vi "Build_footer_text.vi"(4 "Invalid line":string, 6 "Error string":string, 9 "Run time":dbl, 10 "Start time":timestamp, 11 "File Text":string) -> (3 "file w/footer":string)   [LabVIEW 2017, in "labview-standard-library.lvlib" / "automode-scripting.lvlib"]
uses:
  automode-scripting.lvlib
panel:
  out "error out":errorcluster
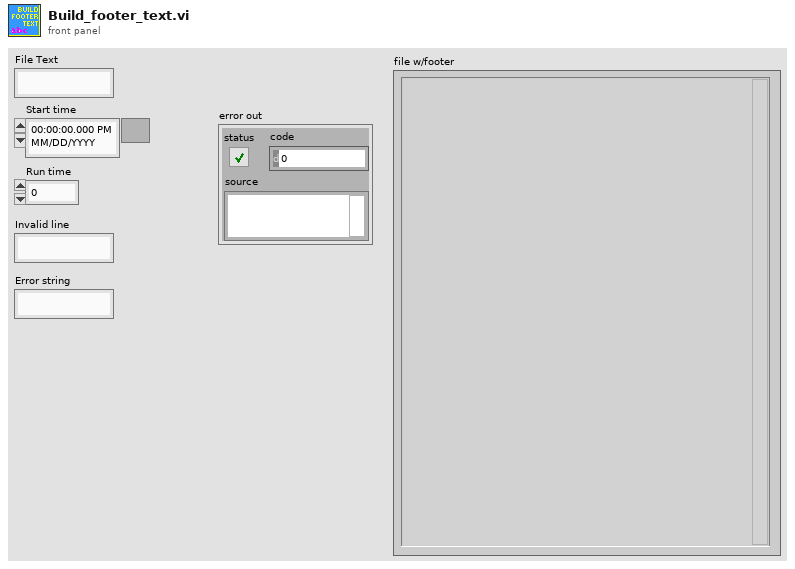
[diagram p1: front panel]
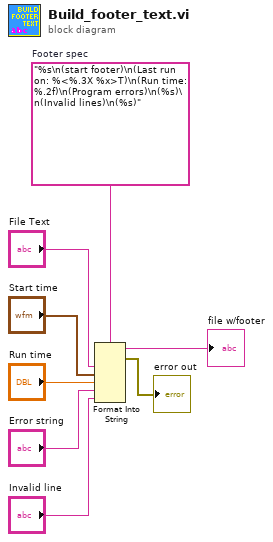
[diagram p0: block diagram]
diagram:
  w1 = "%s\n(start footer)\n(Last run on: %<%.3X %x>T)\n(Run time: %.2f)\n(Program errors)\n(%s)\n(Invalid lines)\n(%s)"  # Footer spec
  n1 = Format Into String(format string=w1, "File Text", "Start time", "Run time", "Error string", "Invalid line") -> (resulting string=→"file w/footer":string, error out=→"error out":errorcluster)  [unwired: 2 in]
